vi "LVIS_SendToDC.vi"(8 "Error In":errorcluster, 11 "Data":string) -> (0 "Error out":errorcluster, 2 "Online?":bool, 3 "TCP Read":string)   [LabVIEW 2015]
doc: "Sends the event data to the Data Commander, allowing for (2) attempts by verifying the response. Writes the data to an error log in the event of failure."
uses:
  Globals/LVIS_DcGlobals.vi
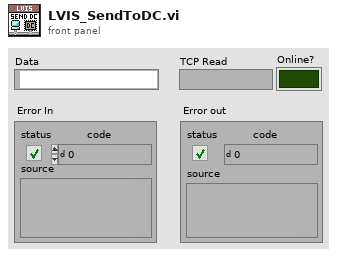
[diagram p1: front panel]
types:
  T1 = enum16{"Standard", "Buffered", "CRLF", "Immediate"}
  T2 = cluster{"ConnTimeout":string, "TxTimeout":string, "RxTimeout":string, "Port":string, "Map":string}
  T3 = cluster{"DCIP":string, "BackupFile":string, "ErrorLog":string, "FilePosition":string}
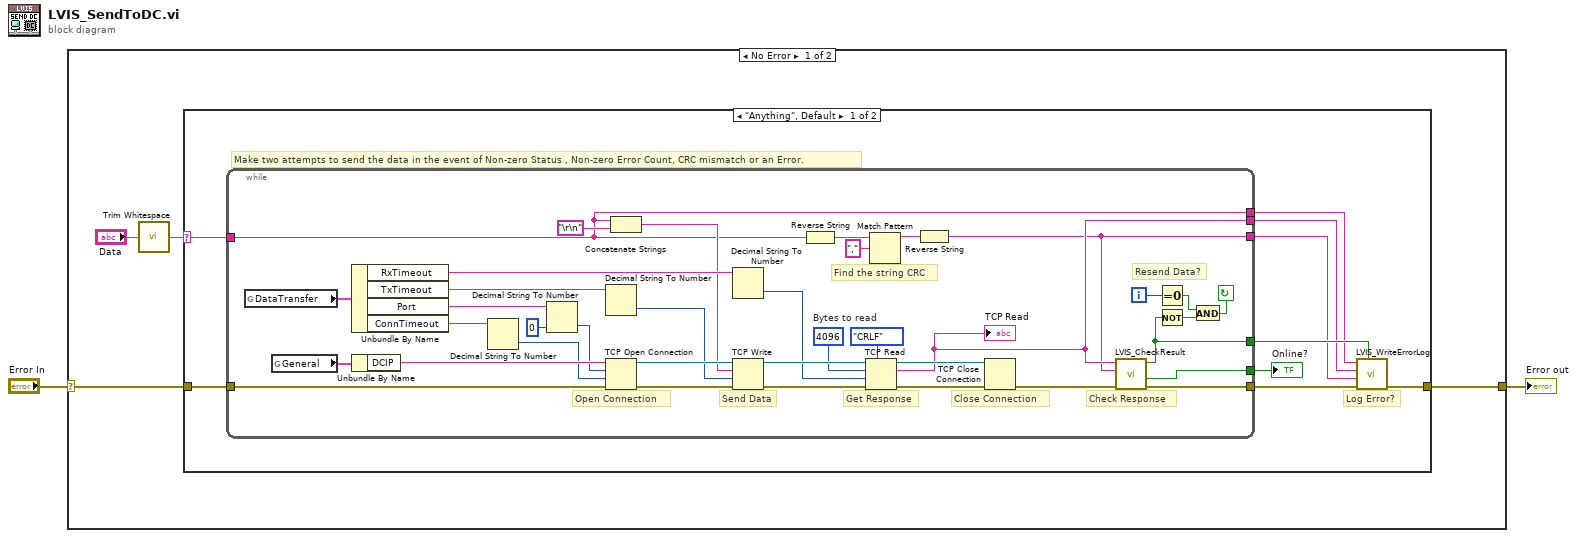
[diagram p0: block diagram]
diagram:
  n1 = case shown="No Error" "Error In" {
    selector: "Error In" -> [w6 w54]
    tunnel: [w5 w54] -> w1
    frame No Error {
      n2 = call <vilib>:"Trim Whitespace.vi"("string"="Data") -> ("trimmed string"=w3:string)  [unwired: 1 in]
      n3 = case shown="\"Anything\", Default" w3 {
        selector: w3 -> [w8 _]
        tunnel: w6 -> [w15 w53]
        tunnel: [w12 w53] -> w5
        frame "Anything", Default {
          # "Make two attempts to send the data in the event of Non-zero Status , Non-zero Error Count, CRC mismatch or an Error."
          # "Log Error?"
          n4 = while {
            tunnel: [w24] -> w14
            tunnel: w15 -> [w43]
            tunnel: [w26] -> w13
            tunnel: [w20] -> w11
            tunnel: [w17] -> w10
            tunnel: [w18] -> w9
            tunnel: w8 -> [w17]
            tunnel: [w16] -> w7
            i -> [w25]
            stop <- w23 continue-if-true
            w44 = 4096  # Bytes to read
            # "Resend Data?"
            # "Check Response"
            # "Find the string CRC"
            # "Close Connection"
            # "Get Response"
            # "Send Data"
            # "Open Connection"
            n5 = global read "LVIS_DcGlobals.vi" "DataTransfer"() -> (w42:T2)
            n6 = global read "LVIS_DcGlobals.vi" "General"() -> (w41:T3)
            n7 = Unbundle By Name(w42) -> ("RxTimeout"=w51:string, "TxTimeout"=w34:string, "Port"=w39:string, "ConnTimeout"=w38:string)
            n8 = Unbundle By Name(w41) -> ("DCIP"=w40:string)
            n9 = Decimal String To Number(string=w38) -> (number=w37:i32)  [unwired: 2 in, 1 out]
            n10 = Decimal String To Number(string=w39, default (0L)=u16 0 ("remote port or service name")) -> (number=w35:u16)  [unwired: 1 in, 1 out]
            n11 = Decimal String To Number(string=w34) -> (number=w33:i32)  [unwired: 2 in, 1 out]
            n12 = TCP Open Connection(address=w40, remote port or service name=w35, timeout ms (60000)=w37, error in (no error)=w43) -> (connection ID=w47:refnum<k5>, error out=w46:errorcluster)  [unwired: 1 in]
            n13 = Concatenate Strings(w17, "\r\n") -> (w19:string)
            n14 = Decimal String To Number(string=w51) -> (number=w32:i32)  [unwired: 2 in, 1 out]
            n15 = TCP Write(connection ID=w47, data in=w19, error in (no error)=w46, 9:w33) -> (connection ID out=w48:refnum<k5>, error out=w52:errorcluster)  [unwired: 1 out]
            n16 = Reverse String(1:w17) -> (0:w29:string)
            n17 = TCP Read(connection ID=w48, bytes to read=w44, error in (no error)=w52, 7:T1."CRLF" ("mode (standard)"), 9:w32) -> (connection ID out=w50:refnum<k5>, data out=w18:string, error out=w49:errorcluster)
            "TCP Read" <- w18
            n18 = Match Pattern(string=w29, regular expression=",") -> (before substring=w27:string)  [unwired: 1 in, 3 out]
            n19 = Reverse String(1:w27) -> (0:w16:string)
            n20 = TCP Close Connection(connection ID=w50, error in (no error)=w49) -> (error out=w30:errorcluster)  [unwired: 1 in, 1 out]
            n21 = call "LVIS_CheckResult.vi"("Error In"=w30, "CRC"=w16, "Response"=w18) -> ("Error out"=w26:errorcluster, "Online?"=w24:bool, "Success?"=w20:bool)  [unwired: 5 in, 1 out]
            n22 = Equal To 0?(x=w25) -> (x = 0?=w21:bool)
            n23 = Not(x=w20) -> (.not. x?=w22:bool)
            n24 = And(x=w21, y=w22) -> (x .and. y?=w23:bool)
          }
          "Online?" <- w14
          n25 = call "LVIS_WriteErrorLog.vi"("Success?"=w11, "Error In"=w13, "Send CRC"=w7, "DC Recieved"=w9, "DC Sent"=w10) -> ("Error out"=w12:errorcluster)  [unwired: 6 in]
        }
        frame "" {
          # "Data is blank or empty, don't attempt to send to the Data Commander"
        }
      }
    }
    frame Error {
    }
  }
  "Error out" <- w1
